vi "imaqio_Open.vi"(0 "Resource Name":T1, 5 "Target Specific String":string, 11 "error in (no error)":errorcluster) -> (4 "Device Handle Out":T2, 15 "error out":errorcluster)   [LabVIEW 2017]
uses:
  <vilib>/LabVIEW Targets/FPGA/RIO/nirio_driverPrimitives.llb/_nirio_device_handleType.ctl
  <vilib>/userdefined/High Color/nirio_resource_hc.ctl
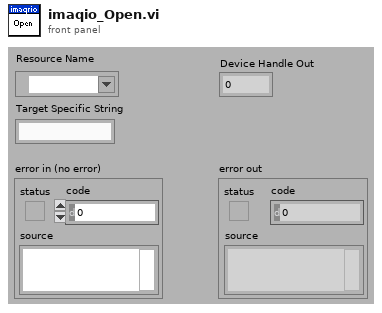
[diagram p1: front panel]
types:
  T1 = typedef "nirio_resource_hc.ctl" = tag
  T2 = typedef "_nirio_device_handleType.ctl" = u32
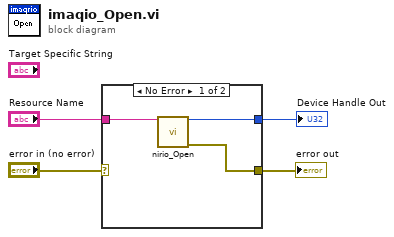
[diagram p0: block diagram]
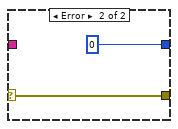
[diagram p2: hidden frame]
diagram:
  n1 = case shown="No Error" "error in (no error)" {
    selector: "error in (no error)" -> [_ w9]
    tunnel: [w5 w9] -> w4
    tunnel: [w6 T2 0 ("Device Handle Out")] -> w2
    tunnel: "Resource Name" -> [w7 _]
    frame No Error {
      n2 = call <vilib>:"nirio_Open.vi"("resource name"=w7) -> ("handle out"=w6:T2, "error out"=w5:errorcluster)  [unwired: 2 in, 11 out]
    }
    frame Error {
    }
  }
  "error out" <- w4
  "Device Handle Out" <- w2
